vi "Enable Card reader.vi"(8 "error in (no error)":errorcluster, 10 "Disabled":T1(ring), 11 "Sim User Console Actor in":refnum<class "Sim User Console Actor.lvclass">) -> (0 "error out":errorcluster, 3 "Sim User Console Actor out":refnum<class "Sim User Console Actor.lvclass">)   [LabVIEW 2019, in "Sim User Console Actor.lvlib" / "Sim User Console Actor.lvclass"]
uses:
  Sim User Console Actor.lvclass
  Sim User Console Actor.lvclass/Sim User Console Actor.ctl
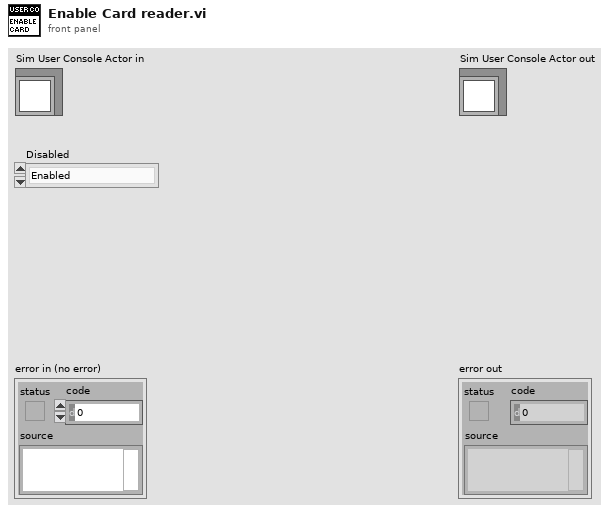
[diagram p1: front panel]
types:
  T1 = enum8{"Enabled", "Disabled", "Disabled and Grayed Out"}
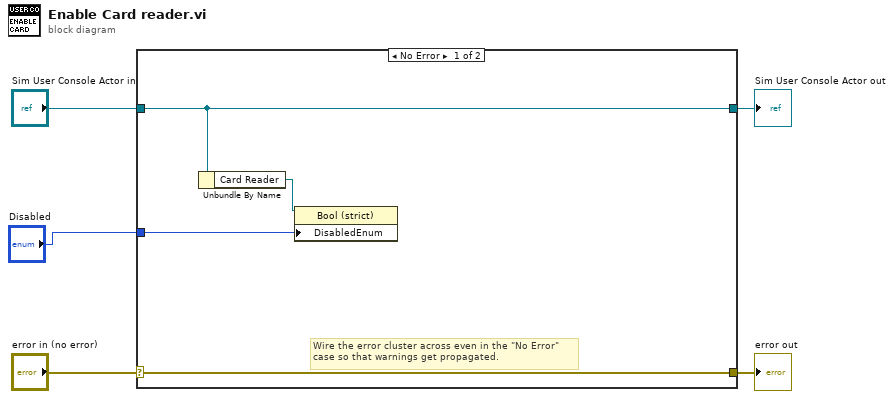
[diagram p0: block diagram]
diagram:
  n1 = case shown="No Error" "error in (no error)" {
    selector: "error in (no error)" -> [w9 w11]
    tunnel: [w9 w11] -> w4
    tunnel: [w8 w10] -> w2
    tunnel: "Sim User Console Actor in" -> [w8 w10]
    tunnel: "Disabled" -> [w6 _]
    frame No Error {
      # "Wire the error cluster across even in the \"No Error\"\ncase so that warnings get propagated."
      n2 = Unbundle By Name(w8) -> ("Card Reader"=w7:refnum<vi>)
      n3 = property class="Bool (strict)"(reference=w7, "DisabledEnum"=w6) -> ()  [unwired: 1 in, 2 out]
    }
    frame Error {
    }
  }
  "error out" <- w4
  "Sim User Console Actor out" <- w2
